vi "WinHostToFlexRIO.vi"() -> ()   [LabVIEW 2013]
uses:
  <vilib>/userdefined/High Color/nirio_resource_hc.ctl
  <vilib>/FPGAPlugInAG/PXIe-7966R/niLvFpga_Open_PXIe-7966R.vi
  <vilib>/FPGAPlugInAG/PXIe-7966R/niLvFpga_Reset_PXIe-7966R.vi
  <vilib>/Utility/error.llb/Error Cluster From Error Code.vi
  <vilib>/rvi/errors/niLvFpgaAdjustHostInterfaceError.vi
  <vilib>/FPGAPlugInAG/PXIe-7966R/niLvFpga_Run_PXIe-7966R.vi
  <vilib>/rvi/interface/common/niFpgaWaitOnOcc.vi
  <vilib>/FPGAPlugInAG/PXIe-7966R/niLvFpga_Close_PXIe-7966R.vi
  <vilib>/rvi/interface/nirviOpenFPGA/nirviOpenFPGA.xnode
  FPGA Bitfiles/PXIe-7966R_FlexRIOMod6581_v1_1.lvbitx
  <vilib>/rvi/interface/nirviMethod/nirviMethod.xnode
  <vilib>/rvi/interface/nirviReadWriteControl/nirviReadWriteControl.xnode
  Control 1.ctl
  <vilib>/rvi/interface/nirviCloseFPGA/nirviCloseFPGA.xnode
  <vilib>/rvi/errors/niLvFpgaMergeErrorWithErrorCode.vi
  NiFpgaLv.dll
  <vilib>/FPGAPlugInAG/PXIe-7966R/niLvFpga_ConfigureFifo_PXIe-7966R.vi
  <vilib>/FPGAPlugInAG/PXIe-7966R/niLvFpga_StartFifo_PXIe-7966R.vi
  <vilib>/FPGAPlugInAG/PXIe-7966R/niLvFpga_ReadFifo_PXIe-7966R.vi
panel:
  in  "DO7":bool
  in  "DO4":bool
  in  "DO2":bool
  out "DI7":bool
  out "DI4":bool
  out "DI2":bool
  out "DI6":bool
  out "DI5":bool
  out "DI3":bool
  in  "DO6":bool
  in  "DO5":bool
  in  "DO3":bool
  in  "auxDO6":bool
  out "DI1":bool
  out "DI0":bool
  in  "DO1":bool
  in  "DO0":bool
  in  "FlexRIO device":T1
  out "DMA0 output":dynamicdata(graph)
  in  "SGSignalType0":enum16{"DC", "Sine", "Square", "Triangle"}(ring)
  in  "stop":bool
  out "SGNo":u8
  in  "SGAmp0":u16
  in  "SamplingRate0":u32=10000
  in  "DMATtoHOSTEnable0":bool
  in  "AO0":i16
  in  "SGFreq0":u32
  in  "SGPhase0":u32
  in  "SGUpdateRate0":u32=10000000
  in  "AOEnable0":bool
  in  "DebugMode":bool
  in  "DAQStartStop":bool
  out "error out":errorcluster
  out "DMATtoHOSTBlockNWords":u16[](array[numeric])
  out "DMATtoHOSTSampleSize":u8[](array[numeric])
  out "DMATtoHOSTNCh":u16[](array[numeric])
  out "DMATtoHOSTFrameType":u8[](array[numeric])
  out "DevProfile":u8
  out "DevTemp":i16
  out "DevQualityStatus":u8
  out "Fref":u32
  out "RIOAdapterCorrect":bool
  out "Expected IO Module ID":u32
  out "InsertedIOModule ID":u32
  out "FPGAVIversion":u8[](array[numeric])
  out "Platform":enum8{"FlexRIO", "cRIO", "RSeries"}(ring)
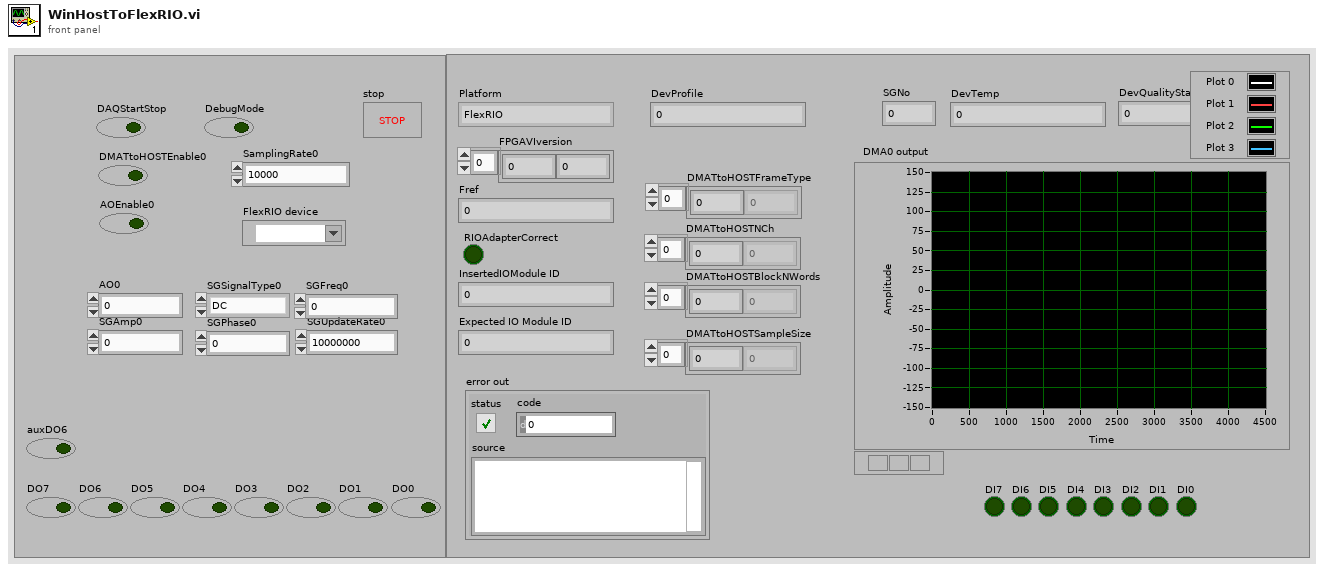
[diagram p1: front panel]
types:
  T1 = typedef "nirio_resource_hc.ctl" = tag
  T2 = enum16{"DAQ-CPU", "IMAQ-CPU", "DAQ-GPU", "IMAQ-GPU"}
  T3 = typedef "Control 1.ctl" = u16
  T4 = cluster{"Timeout":u8, "Timeout":T3, "Timeout":u8, "Timeout":u16}
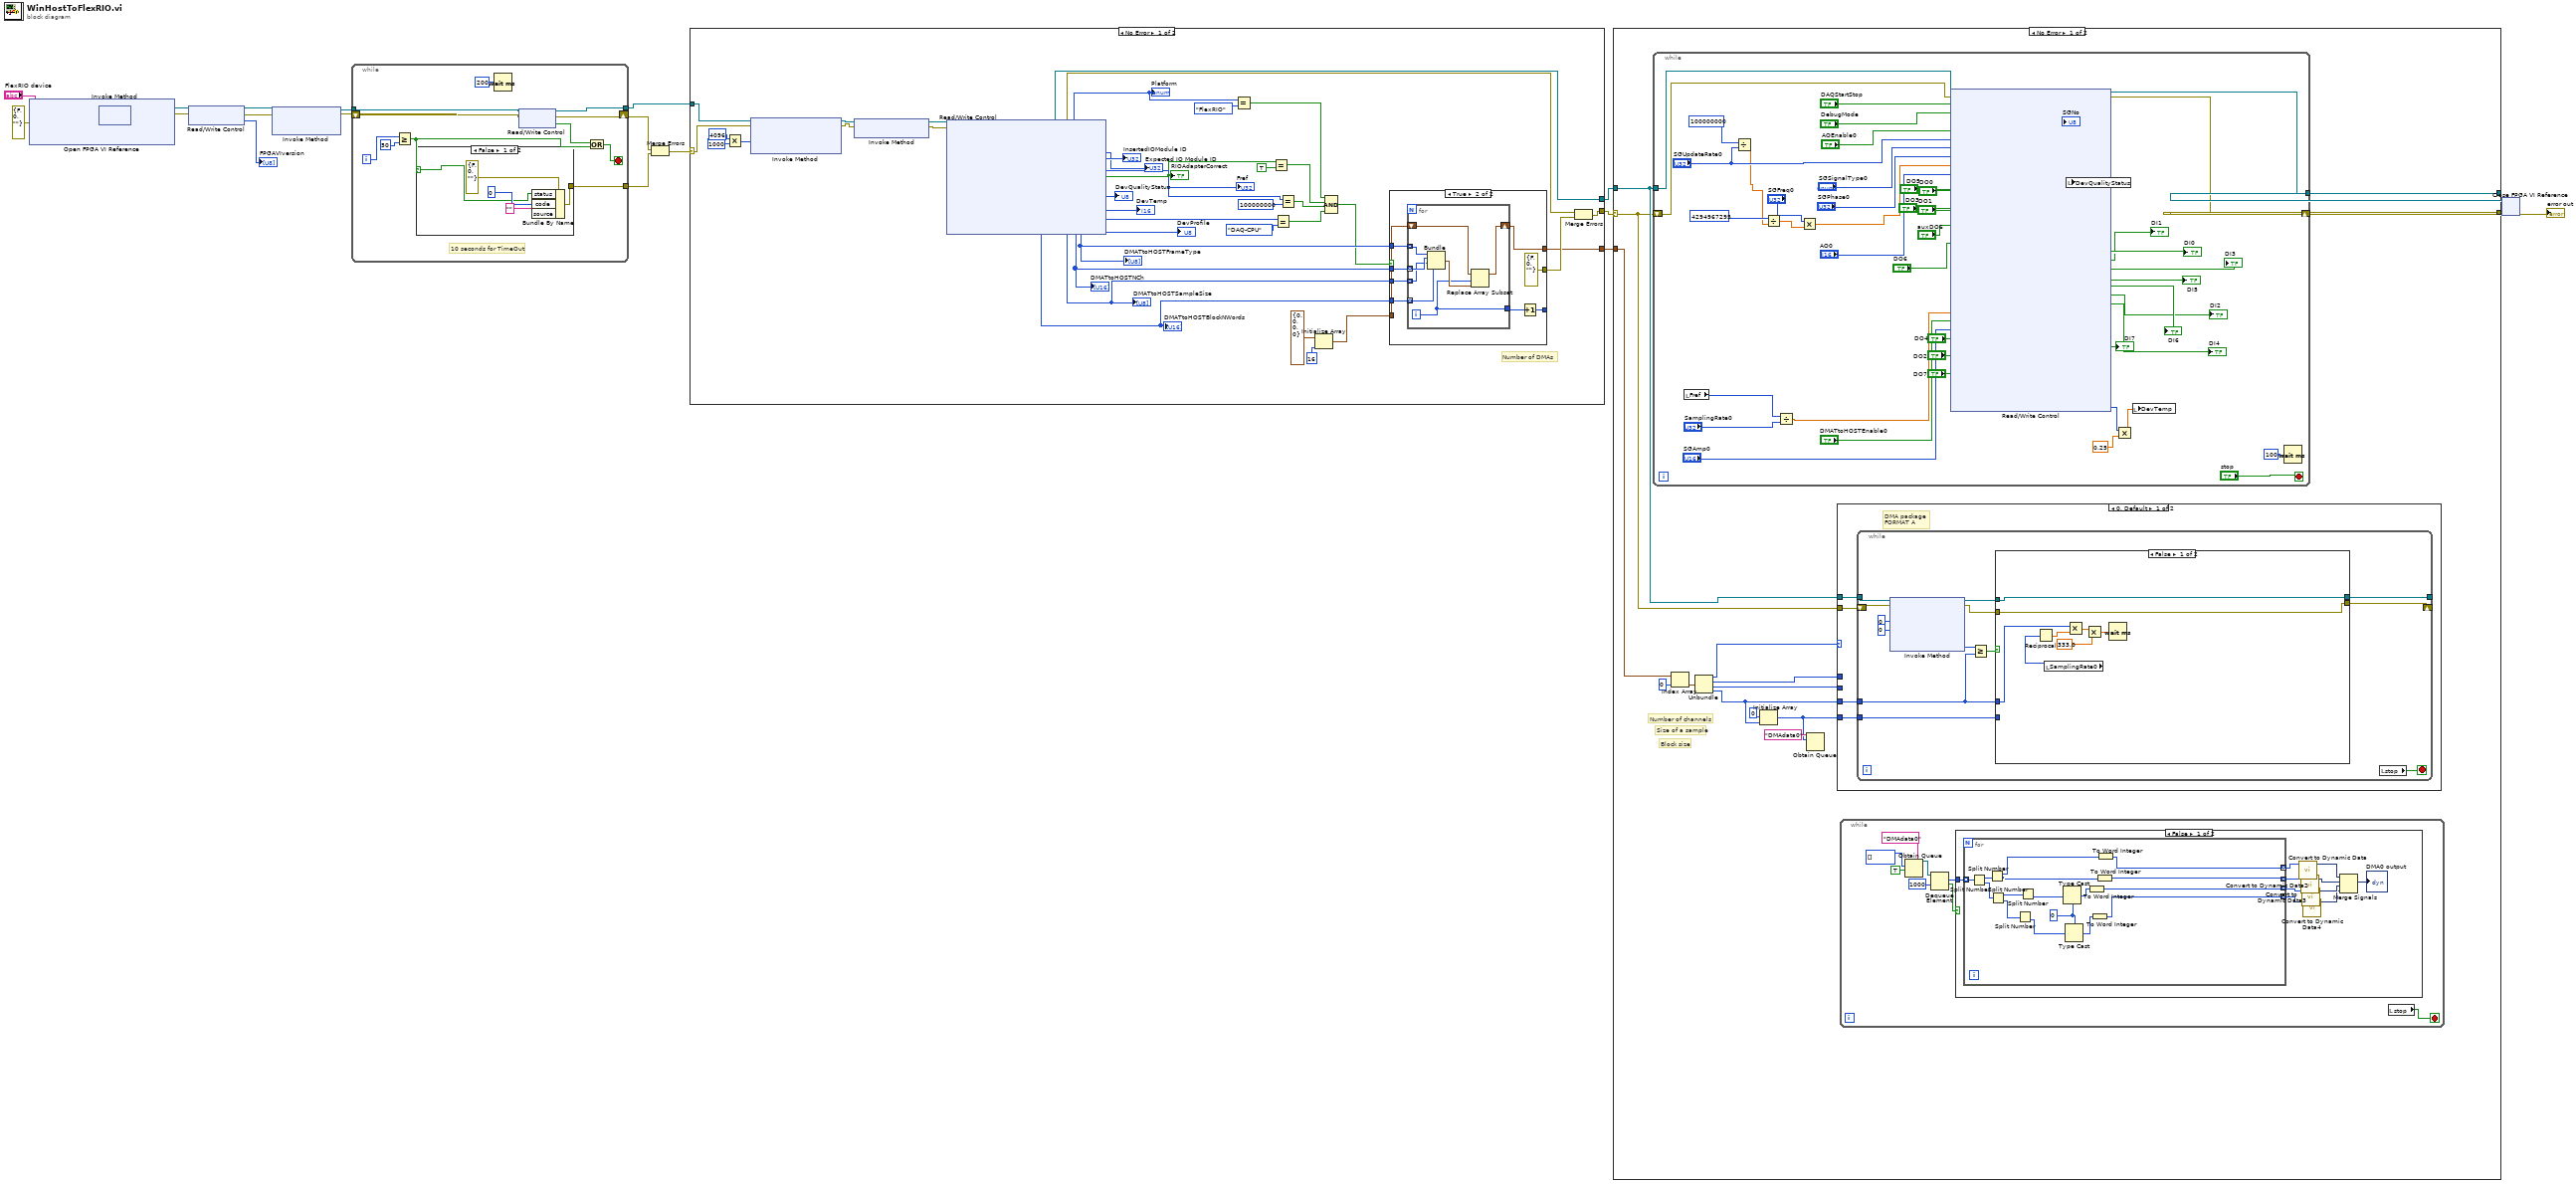
[diagram p0: block diagram]
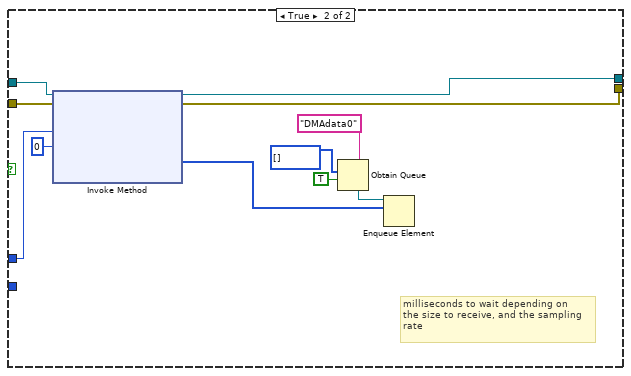
[diagram p3: hidden frame]
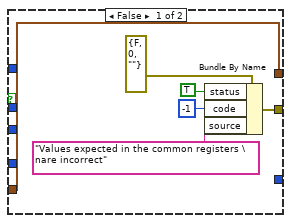
[diagram p6: hidden frame]
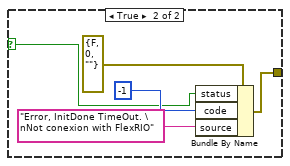
[diagram p8: hidden frame]
diagram:
  n1 = xnode "Open FPGA VI Reference"("error in"=errorcluster {"status"=FALSE, "code"=0, "source"=""}, "resource name"="FlexRIO device") -> ("FPGA VI Reference Out"=w20:refnum<k20>, "error out"=w21:errorcluster)
  n2 = xnode "Invoke Method"("FPGA VI Reference In"=w20, "error in"=w21) -> ("FPGA VI Reference Out"=w5:refnum<k20>, "error out"=w4:errorcluster)
  n3 = xnode "Read/Write Control"("FPGA VI Reference In"=w5, "error in"=w4) -> ("FPGA VI Reference Out"=w3:refnum<k20>, "error out"=w2:errorcluster, "FPGAVIversion"=→"FPGAVIversion":u8[])
  n4 = xnode "Invoke Method"("FPGA VI Reference In"=w3, "error in"=w2) -> ("FPGA VI Reference Out"=w18:refnum<k20>, "error out"=w17:errorcluster)  [unwired: 1 in]
  n5 = while {
    tunnel: w18 -> [w32]
    tunnel: [w29] -> w16
    shift-right: [w30] -> w14
    shift-left: w17 -> [w31]
    tunnel: [w22] -> w15
    i -> [w27]
    stop <- w24 stop-if-true
    # "10 seconds for TimeOut"
    n6 = Greater Or Equal?(x=w27, y=50) -> (x >= y?=w23:bool)
    n7 = case shown="False" w23 {
      selector: w23 -> [w34 w39]
      tunnel: [w33 w38] -> w22
      frame False {
        n8 = Bundle By Name(cluster=errorcluster {"status"=FALSE, "code"=0, "source"=""} ("error constant"), "status"=w34, "code"=0, "source"="") -> (w33:errorcluster)
      }
      frame True {
        n9 = Bundle By Name(cluster=errorcluster {"status"=FALSE, "code"=0, "source"=""} ("error constant"), "status"=w39, "code"=-1, "source"="Error, InitDone TimeOut. \nNot conexion with FlexRIO") -> (w38:errorcluster)
      }
    }
    n10 = Wait (ms)(milliseconds to wait=u32 200) -> ()  [unwired: 1 out]
    n11 = xnode "Read/Write Control"("FPGA VI Reference In"=w32, "error in"=w31) -> ("FPGA VI Reference Out"=w29:refnum<k20>, "error out"=w30:errorcluster, "InitDone"=w25:bool)
    n12 = Or(x=w25, y=w23) -> (x .or. y?=w24:bool)
  }
  n13 = Merge Errors(w14, w15) -> (w13:errorcluster)
  n14 = case shown="No Error" w13 {
    selector: w13 -> [w74 w105]
    tunnel: w16 -> [w75 w104]
    tunnel: [w69 w104] -> w10
    tunnel: [w46 w105] -> w11
    tunnel: [w44 _] -> w7
    frame No Error {
      # "Number of DMAs"
      n15 = Multiply(x=u32 4096 ("Requested Depth"), y=u32 1000) -> (x*y=w76:u32)
      n16 = xnode "Invoke Method"("FPGA VI Reference In"=w75, "error in"=w74, "Requested Depth"=w76) -> ("FPGA VI Reference Out"=w80:refnum<k20>, "error out"=w79:errorcluster)  [unwired: 1 out]
      n17 = xnode "Invoke Method"("FPGA VI Reference In"=w80, "error in"=w79) -> ("FPGA VI Reference Out"=w72:refnum<k20>, "error out"=w73:errorcluster)
      n18 = xnode "Read/Write Control"("FPGA VI Reference In"=w72, "error in"=w73) -> ("FPGA VI Reference Out"=w69:refnum<k20>, "error out"=w47:errorcluster, "Platform"=w68:enum8{"FlexRIO", "cRIO", "RSeries"}, "InsertedIOModule ID"=→"InsertedIOModule ID":u32, "Expected IO Module ID"=→"Expected IO Module ID":u32, "RIOAdapterCorrect"=w64:bool, "Fref"=w66:u32, "DevQualityStatus"=→"DevQualityStatus":u8, "DevTemp"=→"DevTemp":i16, "DevProfile"=w60:u8, "DMATtoHOSTFrameType"=w55:u8[], "DMATtoHOSTNCh"=w58:T3[], "DMATtoHOSTSampleSize"=w57:u8[], "DMATtoHOSTBlockNWords"=w56:u16[])
      "Platform" <- w68
      "RIOAdapterCorrect" <- w64
      "Fref" <- w66
      "DevProfile" <- w60
      "DMATtoHOSTFrameType" <- w55
      "DMATtoHOSTNCh" <- w58
      "DMATtoHOSTSampleSize" <- w57
      "DMATtoHOSTBlockNWords" <- w56
      n19 = Equal?(x=w68, y=enum16{"FlexRIO", "cRIO", "R-Series"}."FlexRIO") -> (x = y?=w43:bool)
      n20 = Equal?(x=w64, y=TRUE) -> (x = y?=w53:bool)
      n21 = Equal?(x=w60, y=T2."DAQ-CPU") -> (x = y?=w51:bool)
      n22 = Equal?(x=w66, y=u32 100000000) -> (x = y?=w52:bool)
      n23 = Initialize Array(cluster{u8, u16, u8, u16} {0, 0, 0, 0}, 16 ("dimension size")) -> (w48:cluster{u8, u16, u8, u16}[])
      n24 = Compound Arithmetic op=AND(w43, w53, w52, w51) -> (w54:bool)
      n25 = case shown="True" w54 {
        tunnel: w58 -> [_ w95]
        tunnel: w57 -> [_ w94]
        tunnel: w56 -> [_ w93]
        tunnel: w55 -> [_ w92]
        tunnel: w48 -> [w81 w91]
        tunnel: [w81 w90] -> w44
        tunnel: [w82 errorcluster {"status"=FALSE, "code"=0, "source"=""} ("error constant")] -> w45
        tunnel: [_ w87] -> _
        frame False {
          n26 = Bundle By Name(cluster=errorcluster {"status"=FALSE, "code"=0, "source"=""} ("error constant"), "status"=TRUE, "code"=-1, "source"="Values expected in the common registers \nare incorrect") -> (w82:errorcluster)
        }
        frame True {
          n27 = for {
            tunnel: w95 -> [w101] mode=indexing
            tunnel: w94 -> [w100] mode=indexing
            tunnel: w93 -> [w99] mode=indexing
            tunnel: w92 -> [w102] mode=indexing
            shift-right: [w97] -> w90
            shift-left: w91 -> [w103]
            tunnel: [w96] -> w88
            i -> [w96]
            n28 = Bundle("Timeout"=w102, "Timeout"=w101, "Timeout"=w100, "Timeout"=w99) -> (w98:T4)  [unwired: 1 in]
            n29 = Replace Array Subset(array=w103, new element=w98, index=w96) -> (w97:cluster{u8, u16, u8, u16}[])
          }
          n30 = Increment(x=w88) -> (x+1=w87:i32)
        }
      }
      n31 = Merge Errors(w47, w45) -> (w46:errorcluster)
    }
    frame Error {
    }
  }
  n32 = case shown="No Error" w11 {
    selector: w11 -> [w111 w237]
    tunnel: w10 -> [w112 w236]
    tunnel: [w119 w236] -> w9
    tunnel: [w118 w237] -> w8
    tunnel: w7 -> [w117 _]
    frame No Error {
      # "Block size"
      # "Size of a sample"
      # "Number of channels"
      n33 = while {
        shift-right: [w223] -> w118
        shift-left: w111 -> [w234]
        tunnel: w112 -> [w235]
        tunnel: [w233] -> w119
        stop <- "stop" stop-if-true
        n34 = local read "Fref"() -> (w220:u32)
        n35 = Divide(x=100000000, y="SGUpdateRate0") -> (x/y=w211:dbl)
        n36 = Divide(x=i64 4294967295, y=w211) -> (x/y=w215:dbl)
        n37 = Divide(x=w220, y="SamplingRate0") -> (x/y=w221:dbl)
        n38 = Multiply(x="SGFreq0", y=w215) -> (x*y=w213:dbl)
        n39 = xnode "Read/Write Control"("FPGA VI Reference In"=w235, "error in"=w234, "DAQStartStop"="DAQStartStop", "DebugMode"="DebugMode", "AOEnable0"="AOEnable0", "SGUpdateRate0"="SGUpdateRate0", "SGSignalType0"="SGSignalType0", "SGPhase0"="SGPhase0", "SGFreq0"=w213, "AO0"="AO0", "DO0"="DO0", "DO1"="DO1", "DO3"="DO3", "DO5"="DO5", "auxDO6"="auxDO6", "DO6"="DO6", "DMATtoHOSTSamplingRate0"=w221, "DMATtoHOSTEnable0"="DMATtoHOSTEnable0", "SGAmp0"="SGAmp0", "DO2"="DO2", "DO4"="DO4", "DO7"="DO7") -> ("FPGA VI Reference Out"=w233:refnum<k20>, "error out"=w223:errorcluster, "SGNo"=→"SGNo":u8, "DevQualityStatus"=w224:u8, "DI0"=→"DI0":bool, "DI1"=→"DI1":bool, "DI3"=→"DI3":bool, "DI5"=→"DI5":bool, "DI6"=→"DI6":bool, "DI2"=→"DI2":bool, "DI4"=→"DI4":bool, "DI7"=→"DI7":bool, "DevTemp"=w192:i16)  [unwired: 4 in, 1 out]
        n40 = local write "DevQualityStatus"(w224) -> ()
        n41 = Multiply(x=w192, y=0.25) -> (x*y=w191:dbl)
        n42 = local write "DevTemp"(w191) -> ()
        n43 = Wait (ms)(milliseconds to wait=u32 100) -> ()  [unwired: 1 out]
      }
      n44 = Index Array(array=w117, index=0) -> (element=w115:cluster{u8, u16, u8, u16})
      n45 = Unbundle(w115) -> (w114:u8, w113:u16, w110:u8, w108:u16)
      n46 = Initialize Array(u64 0, w108) -> (w106:u64[])
      n47 = Obtain Queue(name (unnamed)="DMAdata0", element data type=w106) -> ()  [unwired: 3 in, 3 out]
      n48 = case shown="0, Default" w114 {
        tunnel: w113 -> [_ _]
        tunnel: w110 -> [_ _]
        tunnel: w108 -> [w154 _]
        tunnel: w112 -> [w157 _]
        tunnel: w111 -> [w155 _]
        tunnel: w106 -> [w156 _]
        frame 0, Default {
          # "DMA package \nFORMAT A"
          n49 = while {
            tunnel: w157 -> [w167]
            tunnel: w156 -> [w160]
            tunnel: w154 -> [w162]
            tunnel: [w169] -> _
            shift-right: [w168] -> _
            shift-left: w155 -> [w166]
            stop <- w170 stop-if-true
            n50 = xnode "Invoke Method"("FPGA VI Reference In"=w167, "error in"=w166, "Number of Elements"=u32 0, "Timeout (ms)"=0) -> ("FPGA VI Reference Out"=w159:refnum<k20>, "error out"=w158:errorcluster, "Elements Remaining"=w163:u32)  [unwired: 1 out]
            n51 = Greater Or Equal?(x=w163, y=w162) -> (x >= y?=w161:bool)
            n52 = case shown="False" w161 {
              tunnel: [w172 w189] -> w169
              tunnel: [w171 w188] -> w168
              tunnel: w162 -> [w174 w187]
              tunnel: w160 -> [_ _]
              tunnel: w159 -> [w172 w180]
              tunnel: w158 -> [w171 w179]
              frame False {
                n53 = local read "SamplingRate0"() -> (w173:u32)
                n54 = Reciprocal(x=w173) -> (1/x=w178:dbl)
                n55 = Multiply(x=w174, y=w178) -> (x*y=w177:dbl)
                n56 = Multiply(x=w177, y=333.0) -> (x*y=w175:dbl)
                n57 = Wait (ms)(milliseconds to wait=w175) -> ()  [unwired: 1 out]
              }
              frame True {
                # "milliseconds to wait depending on \nthe size to receive, and the sampling\nrate"
                n58 = xnode "Invoke Method"("FPGA VI Reference In"=w180, "error in"=w179, "Number of Elements"=w187, "Timeout (ms)"=0) -> ("FPGA VI Reference Out"=w189:refnum<k20>, "error out"=w188:errorcluster, "Data"=w181:u64[])  [unwired: 1 out]
                n59 = Obtain Queue(name (unnamed)="DMAdata0", element data type=u64[] [], create if not found? (T)=TRUE) -> (queue out=w185:refnum<queue>)  [unwired: 2 in, 2 out]
                n60 = Enqueue Element(queue=w185, element=w181) -> ()  [unwired: 2 in, 3 out]
              }
            }
            n61 = local read "stop"() -> (w170:bool)
          }
        }
        frame 1 {
        }
      }
      n62 = while {
        stop <- w122 stop-if-true
        n63 = Obtain Queue(name (unnamed)="DMAdata0", element data type=u64[] [], create if not found? (T)=TRUE) -> (queue out=w124:refnum<queue>)  [unwired: 2 in, 2 out]
        n64 = Dequeue Element(queue=w124, timeout in ms (-1)=1000) -> (element=w123:u64[], timed out?=w120:bool)  [unwired: 1 in, 2 out]
        n65 = case shown="False" w120 {
          tunnel: w123 -> [w137 _]
          frame False {
            n66 = for {
              tunnel: w137 -> [w153] mode=indexing
              tunnel: [w145] -> w135 mode=indexing
              tunnel: [w147] -> w134 mode=indexing
              tunnel: [w149] -> w133 mode=indexing
              tunnel: [w150] -> w131 mode=indexing
              w139 = i8 0
              n67 = Split Number(x=w153) -> (hi(x)=w152:u32, lo(x)=w151:u32)
              n68 = Split Number(x=w152) -> (hi(x)=w146:u16, lo(x)=w148:u16)
              n69 = Split Number(x=w151) -> (hi(x)=w141:u16, lo(x)=w144:u16)
              n70 = Split Number(x=w144) -> (lo(x)=w143:u8)  [unwired: 1 out]
              n71 = Split Number(x=w141) -> (lo(x)=w140:u8)  [unwired: 1 out]
              n72 = Type Cast(type=w139, x=w140) -> (*(type *) &x=w138:i8)
              n73 = Type Cast(type=w139, x=w143) -> (*(type *) &x=w142:i8)
              n74 = To Word Integer(number=w138) -> (16bit integer=w149:i16)
              n75 = To Word Integer(number=w142) -> (16bit integer=w150:i16)
              n76 = To Word Integer(number=w148) -> (16bit integer=w147:i16)
              n77 = To Word Integer(number=w146) -> (16bit integer=w145:i16)
            }
            n78 = call "Convert to Dynamic Data"("Array"=w135) -> ("Dynamic Data Type"=w128:dynamicdata)  [unwired: 3 in]
            n79 = call "Convert to Dynamic Data2"("Array"=w134) -> ("Dynamic Data Type"=w129:dynamicdata)  [unwired: 3 in]
            n80 = call "Convert to Dynamic Data3"("Array"=w133) -> ("Dynamic Data Type"=w132:dynamicdata)  [unwired: 3 in]
            n81 = call "Convert to Dynamic Data4"("Array"=w131) -> ("Dynamic Data Type"=w130:dynamicdata)  [unwired: 3 in]
            n82 = Merge Signals(w128, w129, w132, w130) -> (→"DMA0 output":dynamicdata)
          }
          frame True {
          }
        }
        n83 = local read "stop"() -> (w122:bool)
      }
    }
    frame Error {
    }
  }
  n84 = xnode "Close FPGA VI Reference"("FPGA VI Reference In"=w9, "error in"=w8) -> ("error out"=→"error out":errorcluster)
